vi "(SubVI)calculate conversion factor and force constant.vi"(3 "X=T\nY=F":bool=TRUE, 5 "laser power (mW)":dbl) -> (0 "conversion factor (V/um)":dbl, 2 "force constant (pN/nm)":dbl)   [LabVIEW 2014]
uses:
  <vilib>/Utility/file.llb/Read From Spreadsheet File (DBL).vi
panel:
  out "Convf-cal-array":dbl[](array[numeric])
  out "Fc-cal-array":dbl[](array[numeric])
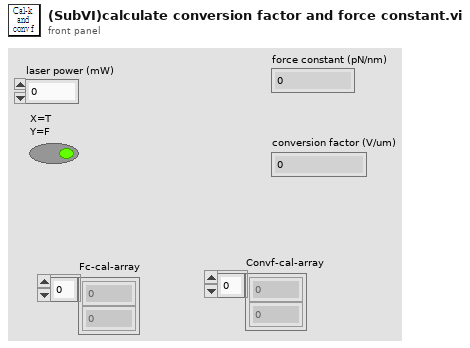
[diagram p1: front panel]
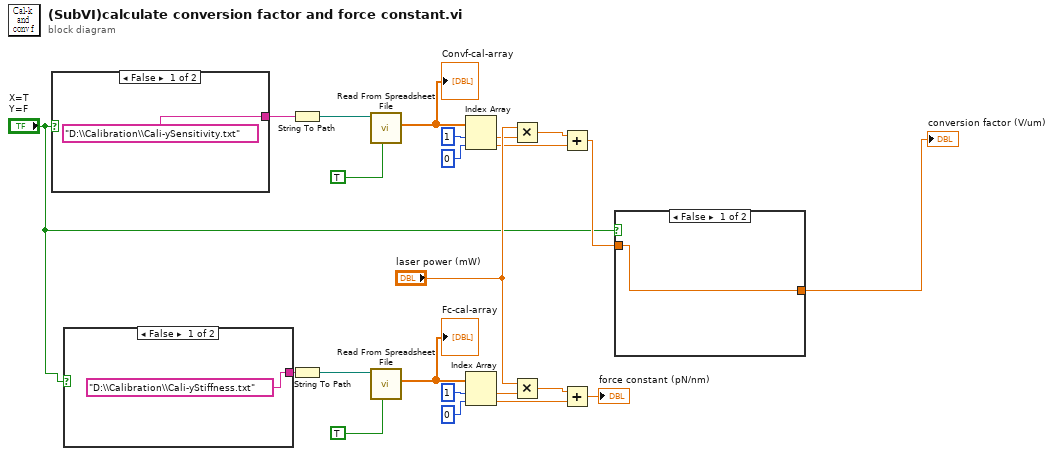
[diagram p0: block diagram]
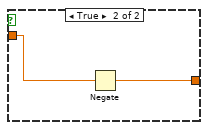
[diagram p2: hidden frame]
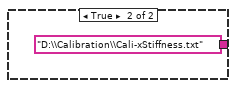
[diagram p3: hidden frame]
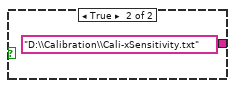
[diagram p4: hidden frame]
diagram:
  n1 = case shown="False" "X=T\nY=F" {
    tunnel: ["D:\\Calibration\\Cali-ySensitivity.txt" "D:\\Calibration\\Cali-xSensitivity.txt"] -> w11
    frame False {
    }
    frame True {
    }
  }
  n2 = case shown="False" "X=T\nY=F" {
    tunnel: ["D:\\Calibration\\Cali-yStiffness.txt" "D:\\Calibration\\Cali-xStiffness.txt"] -> w10
    frame False {
    }
    frame True {
    }
  }
  n3 = String To Path(string=w11) -> (path=w9:path)
  n4 = String To Path(string=w10) -> (path=w8:path)
  n5 = call-poly <vilib>:"Read From Spreadsheet File.vi"("transpose (no:F)"=TRUE, "file path (dialog if empty)"=w9) -> ("first row"=w4:dbl[])  [unwired: 5 in, 4 out]
  "Convf-cal-array" <- w4
  n6 = call-poly <vilib>:"Read From Spreadsheet File.vi"("transpose (no:F)"=TRUE, "file path (dialog if empty)"=w8) -> ("first row"=w5:dbl[])  [unwired: 5 in, 4 out]
  "Fc-cal-array" <- w5
  n7 = Index Array(array=w4, index #1=1 ("index"), index #2=0 ("index")) -> (element #1=w15:dbl, element #2=w14:dbl)
  n8 = Index Array(array=w5, index #1=1 ("index"), index #2=0 ("index")) -> (element #1=w13:dbl, element #2=w12:dbl)
  n9 = Multiply(x="laser power (mW)", y=w15) -> (x*y=w23:dbl)
  n10 = Multiply(x="laser power (mW)", y=w13) -> (x*y=w21:dbl)
  n11 = Add(x=w23, y=w14) -> (x+y=w3:dbl)
  n12 = Add(x=w21, y=w12) -> (x+y=→"force constant (pN/nm)":dbl)
  n13 = case shown="False" "X=T\nY=F" {
    tunnel: w3 -> [w28 w30]
    tunnel: [w28 w29] -> w1
    frame False {
    }
    frame True {
      n14 = Negate(x=w30) -> (-x=w29:dbl)
    }
  }
  "conversion factor (V/um)" <- w1
